vi "Config UserPwd DB.vi"(8 "error in (no error)":errorcluster, 11 "Configuration in":refnum<class "Configuration.lvclass">) -> (0 "error out":errorcluster, 3 "Configuration out":refnum<class "Configuration.lvclass">)   [LabVIEW 2016, in "UserPwd DB.lvlib" / "UserPwd DB Configuration.lvclass"]
uses:
  <userlib>/Common Components/UserPwd DB/UserPwd DB Config/UserPwd DB Configuration.lvclass
  <userlib>/Configuration Dialog Actor/Configuration.lvclass
  <userlib>/Common Components/UserPwd DB/UserPwd DB Config/data row.ctl
  <userlib>/Common Components/UserPwd DB/UserPwd DB Config/Access Level.ctl
  C:/Program Files (x86)/National Instruments/LabVIEW 2016/user.lib/Configuration Dialog Actor/Configuration.lvclass
  <userlib>/Common Components/UserPwd DB/UserPwd DB Config/UserPwd DB Configuration.lvclass/UserPwd DB Configuration.ctl
  <userlib>/Common Components/UserPwd DB/UserPwd DB/Data input.ctl
  <userlib>/Common Components/UserPwd DB/UserPwd DB/Access Level.ctl
  <userlib>/Common Components/UserPwd DB/UserPwd DB/UserPwd DB.lvclass
panel:
  out "Permission Labels":string[](array[string])
  in  "Remove Selected":bool
  in  "New User":bool
  in  "UserPwd Array":T1[](array[typedef]) {"Access Level" items=["Admin"=0, "User"=1, "Guest"=10]}
  in  "Revert":bool
  in  "Apply":bool
  # "Username"
  # "Access Level"
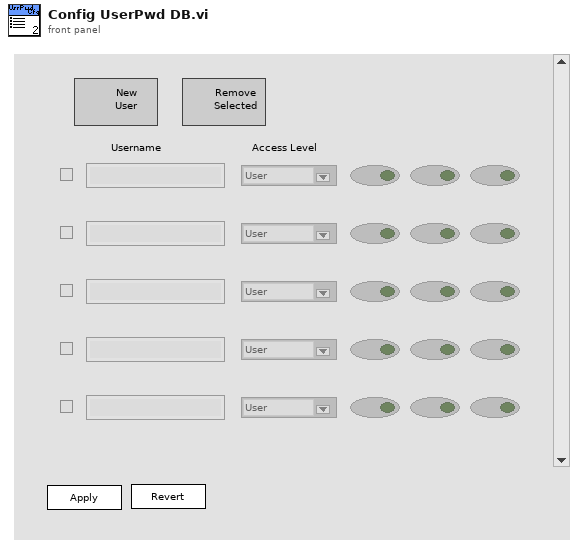
[diagram p1: front panel]
types:
  T1 = typedef "UserPwd DB.lvlib/UserPwd DB Configuration.lvclass/data row.ctl" = cluster{"Checkbox":bool, "Username":string, "Access Level":T2, "Array of Permissions":bool[]}
  T2 = typedef "UserPwd DB.lvlib/UserPwd DB Configuration.lvclass/Access Level.ctl" = u16
  T3 = typedef "UserPwd DB.lvlib/UserPwd DB.lvclass/Data input.ctl" = cluster{"Password":string, "Access":T4, "Array of Permissions":bool[]}
  T4 = typedef "UserPwd DB.lvlib/UserPwd DB.lvclass/Access Level.ctl" = enum16{"Admin", "User lv1", "User lv2", "User lv3", "User lv4", "User lv5", "User lv6", "User lv7", "User lv8", "User lv9", "Guest"}
  T5 = cluster{bool, string, "Access":T4, "2D Array of Permissions":bool[]}
  T6 = cluster{"Checkbox":bool, "Username":bool, "Access Level":bool, "Array of Permissions":bool[]}[]
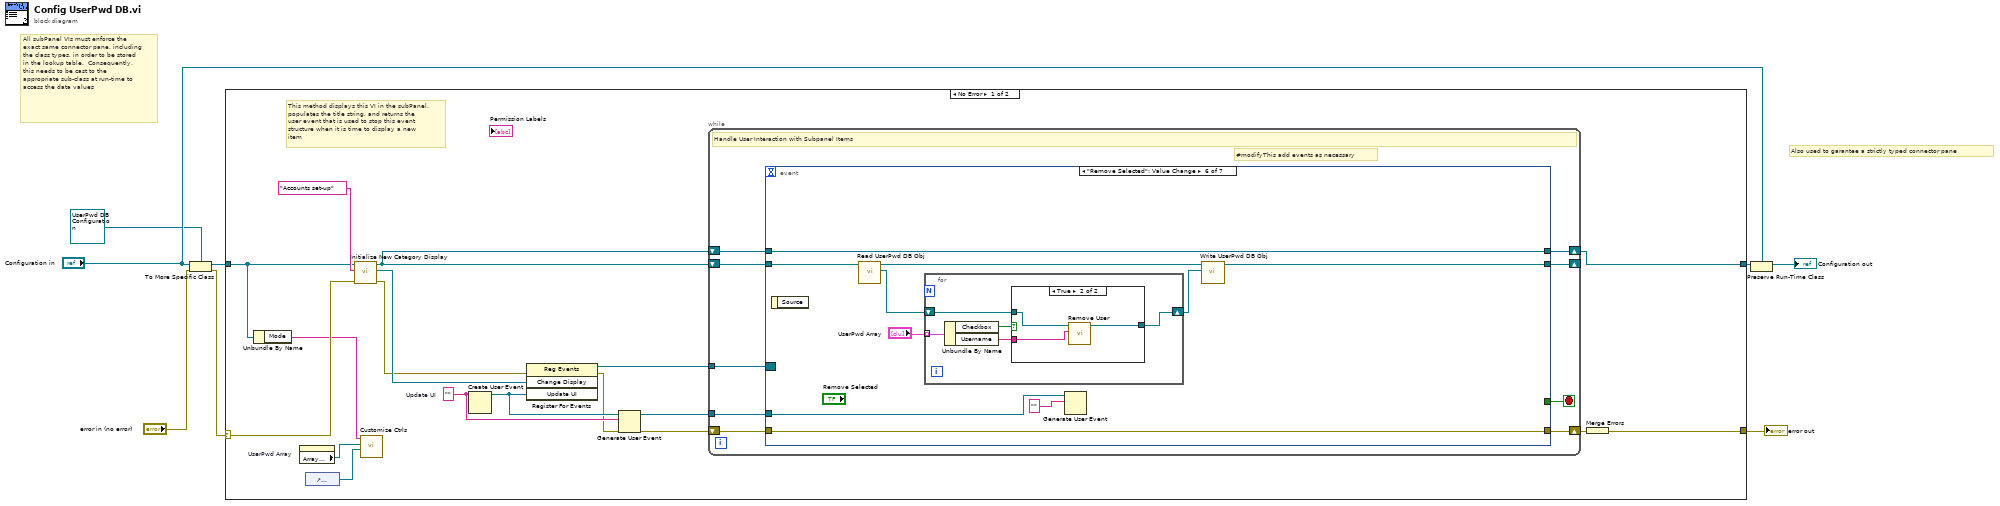
[diagram p0: block diagram]
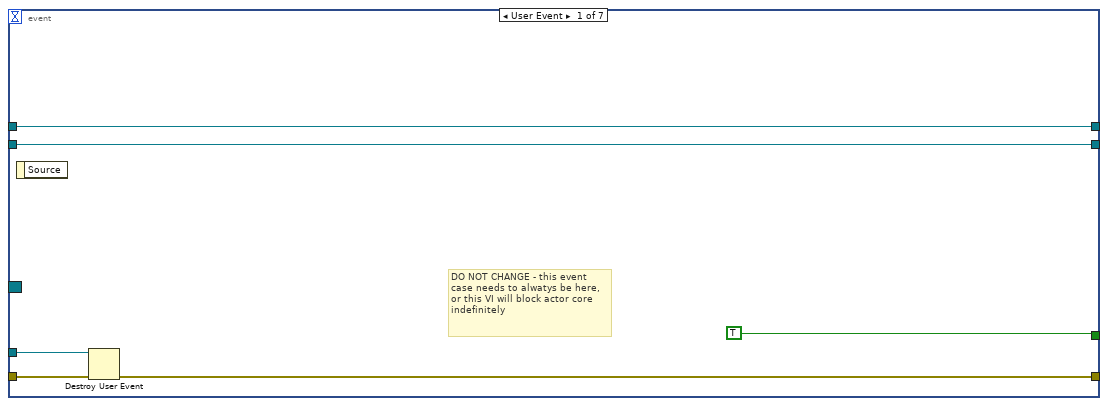
[diagram p2: hidden frame]
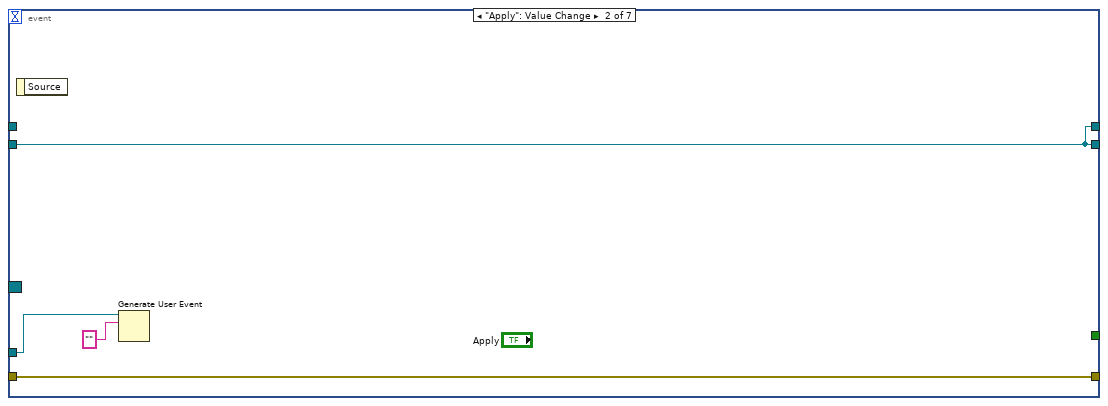
[diagram p3: hidden frame]
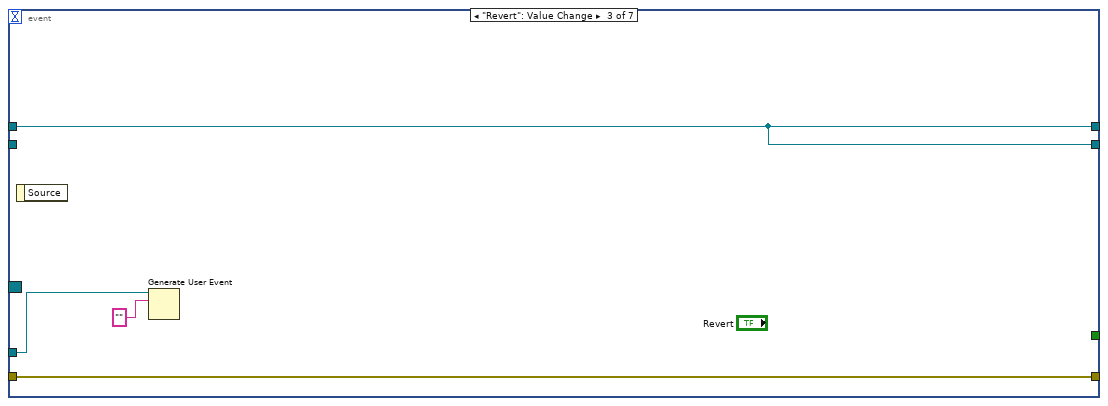
[diagram p4: hidden frame]
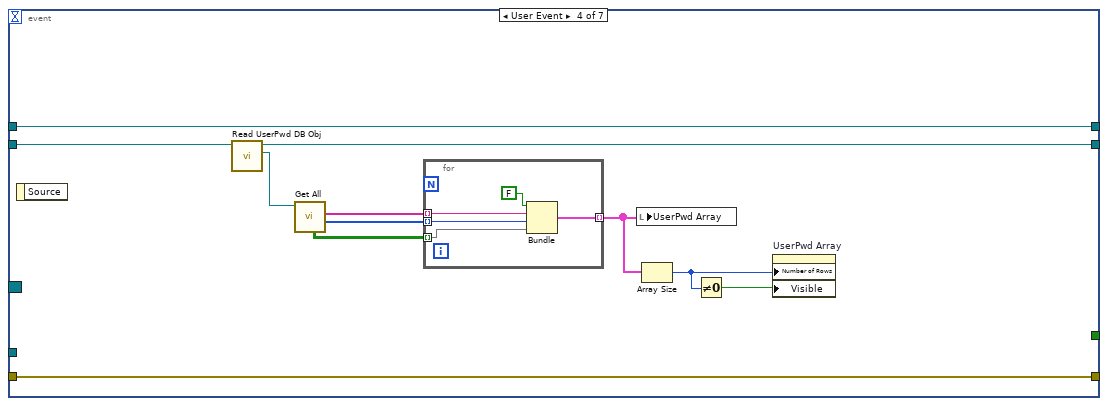
[diagram p5: hidden frame]
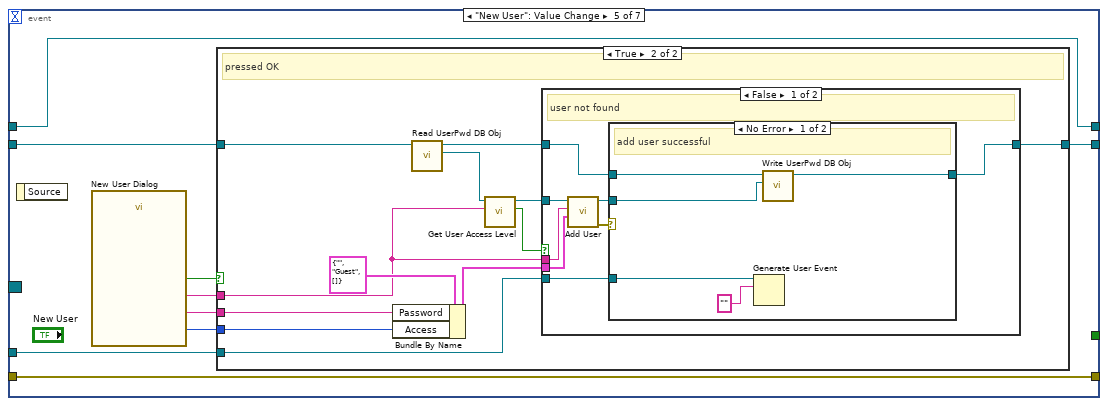
[diagram p6: hidden frame]
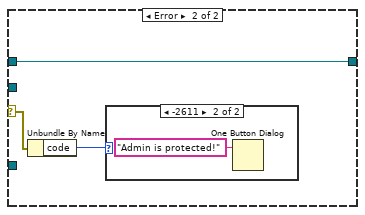
[diagram p8: hidden frame]
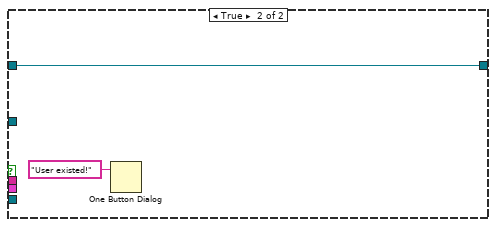
[diagram p10: hidden frame]
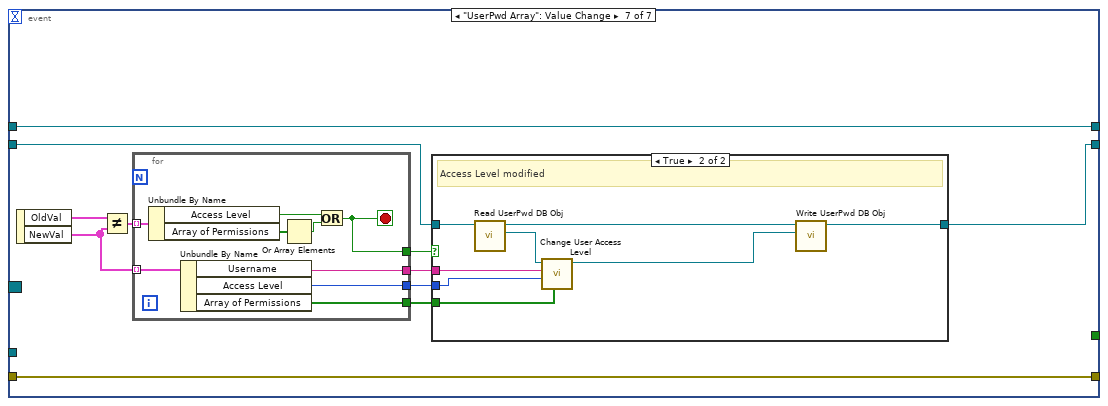
[diagram p12: hidden frame]
diagram:
  # "Also used to garantee a strictly typed connector pane"
  # "All subPanel VIs must enforce the exact same connector pane, including the class types, in order to be stored in the lookup table.  Consequently, this needs to be cast to the appropriate sub-class at run-time to access the data values"
  n1 = To More Specific Class(target class=refnum<class "UserPwd DB Configuration.lvclass"> refnum ("UserPwd DB.lvlib:UserPwd DB Configuration.lvclass"), reference="Configuration in", error in="error in (no error)") -> (specific class reference=w6:refnum<class "UserPwd DB Configuration.lvclass">, error out=w2:errorcluster)
  n2 = case shown="No Error" w2 {
    selector: w2 -> [w24 w155]
    tunnel: w6 -> [w10 w156]
    tunnel: [w17 w156] -> w8
    tunnel: [w26 w155] -> w7
    frame No Error {
      w18 = ""  # Update UI
      # "This method displays this VI in the subPanel, populates the title string, and returns the user event that is used to stop this event structure when it is time to display a new item"
      n3 = Unbundle By Name(w10) -> ("Mode"=w9:string)
      n4 = property on="UserPwd Array" class="Arr (strict)"() -> ("Array Element"=w12:refnum<vi>)  [unwired: 2 in, 2 out]
      n5 = control-ref of="Permission Labels"() -> (w11:refnum<vi>)
      n6 = call <userlib>:"Initialize New Category Display.vi"("error in (no error)"=w24, "Name to Display"="Accounts set-up", "Configuration in"=w10) -> ("error out"=w15:errorcluster, "Change Display"=w23:refnum<user-event>, "Configuration Out"=w20:refnum<class "UserPwd DB Configuration.lvclass">)  [unwired: 6 in]
      n7 = call <userlib>:"Customize Ctrls.vi"("Permission Labels Ref"=w11, "Array Element Ref"=w12, "Mode"=w9) -> ()  [unwired: 8 in, 1 out]
      n8 = Create User Event(user event datatype=w18) -> (user event=w19:refnum<user-event>)  [unwired: 1 in, 1 out]
      n9 = register-events(error in=w15, w23, w19) -> (reference out=w22:refnum<event-registration>, error out=w14:errorcluster)  [unwired: 1 in]
      n10 = Generate User Event(user event=w19, event data cluster=w18, error in=w14) -> (user event out=w16:refnum<user-event>, error out=w13:errorcluster)  [unwired: 1 in]
      n11 = while {
        tunnel: w22 -> [w34]
        shift-right: [w33] -> w21
        shift-left: w13 -> [w32]
        shift-right: [w30] -> _
        shift-left: w20 -> [w31]
        tunnel: w16 -> [w28]
        shift-right: [w27] -> w17
        shift-left: w20 -> [w29]
        stop <- w35 stop-if-true
        # "#modifyThis add events as necessary"
        # "Handle User Interaction with Subpanel Items"
        n12 = event shown="[5] \"Remove Selected\": Value Change" {
          selector: w34 -> [_ _ _ _ _ _ _]
          dyn-events: _ -> [_ _ _ _ _ _ _]
          timeout: _ -> [_ _ _ _ _ _ _]
          tunnel: [TRUE _ _ _ _ _ _] -> w35
          tunnel: [w36 w45 w49 w60 w74 w116 w136] -> w33
          tunnel: w32 -> [w37 w45 w49 w60 w74 w116 w136]
          tunnel: w31 -> [w40 w44 _ w59 w71 w115 w131]
          tunnel: [w40 w44 w48 w58 w72 w110 w130] -> w30
          tunnel: w29 -> [w39 _ w48 w54 w66 w114 w135]
          tunnel: w28 -> [w38 w42 w46 _ w67 w108 _]
          tunnel: [w39 w44 w48 w54 w66 w114 w135] -> w27
          event User Event {
            # "DO NOT CHANGE - this event case needs to alwatys be here, or this VI will block actor core indefinitely"
            n13 = event-data() -> ()  [unwired: 1 in, 1 out]
            n14 = Destroy User Event(user event=w38, error in=w37) -> (error out=w36:errorcluster)
          }
          event "Apply": Value Change {
            n15 = event-data() -> ()  [unwired: 1 in, 1 out]
            n16 = Generate User Event(user event=w42, event data cluster="" ("event data")) -> ()  [unwired: 2 in, 2 out]
          }
          event "Revert": Value Change {
            n17 = event-data() -> ()  [unwired: 1 in, 1 out]
            n18 = Generate User Event(user event=w46, event data cluster="" ("event data")) -> ()  [unwired: 2 in, 2 out]
          }
          event User Event {
            n19 = event-data() -> ()  [unwired: 1 in, 1 out]
            n20 = call <userlib>:"Read UserPwd DB Obj.vi"("UserPwd DB Configuration in"=w59) -> ("UserPwd DB.lvlib:UserPwd DB.lvclass"=w55:refnum<class "UserPwd DB.lvclass">, "UserPwd DB Configuration out"=w58:refnum<class "UserPwd DB Configuration.lvclass">)  [unwired: 9 in]
            n21 = call <userlib>:"Get All.vi"("UserPwd DB in"=w55) -> ("Access Levels"=w56:T4[], "Usernames"=w57:string[], "2D Array of Permissions"=w50:bool[][])  [unwired: 6 in, 2 out]
            n22 = for {
              tunnel: w57 -> [w65] mode=indexing
              tunnel: w56 -> [w64] mode=indexing
              tunnel: [w63] -> w53 mode=indexing
              tunnel: w50 -> [w61] mode=indexing
              n23 = Bundle(FALSE, w65, "Access"=w64, "2D Array of Permissions"=w61) -> (w63:T5)  [unwired: 1 in]
            }
            n24 = local write "UserPwd Array"(w53) -> ()
            n25 = Array Size(array=w53) -> (size(s)=w52:i32)
            n26 = Not Equal To 0?(x=w52) -> (x != 0?=w51:bool)
            n27 = property on="UserPwd Array" class="Arr (strict)"("Number of Rows"=w52, "Visible"=w51) -> ()  [unwired: 2 in, 2 out]
          }
          event "New User": Value Change {
            n28 = event-data() -> ()  [unwired: 1 in, 1 out]
            n29 = call <userlib>:"New User Dialog.vi"() -> ("Access Level"=w70:T2, "Password"=w69:string, "Username"=w68:string, "OK"=w73:bool)  [unwired: 15 in, 1 out]
            n30 = case shown="True" w73 {
              tunnel: [w75 w76] -> w72
              tunnel: w71 -> [w75 w87]
              tunnel: w70 -> [_ w84]
              tunnel: w69 -> [_ w82]
              tunnel: w68 -> [_ w79]
              tunnel: w67 -> [_ w78]
              frame False {
              }
              frame True {
                # "pressed OK"
                n31 = Bundle By Name(cluster=T3 {"Password"="", "Access"=enum."Guest", "Array of Permissions"=[]} ("Data"), "Password"=w82, "Access"=w84) -> (w83:T3)
                n32 = call <userlib>:"Read UserPwd DB Obj.vi"("UserPwd DB Configuration in"=w87) -> ("UserPwd DB.lvlib:UserPwd DB.lvclass"=w86:refnum<class "UserPwd DB.lvclass">, "UserPwd DB Configuration out"=w77:refnum<class "UserPwd DB Configuration.lvclass">)  [unwired: 9 in]
                n33 = call <userlib>:"Get User Access Level.vi"("Username"=w79, "UserPwd DB in"=w86) -> ("found"=w80:bool, "UserPwd DB out"=w81:refnum<class "UserPwd DB.lvclass">)  [unwired: 5 in, 3 out]
                n34 = case shown="False" w80 {
                  tunnel: w83 -> [w95 _]
                  tunnel: w79 -> [w94 _]
                  tunnel: w81 -> [w93 _]
                  tunnel: w78 -> [w92 _]
                  tunnel: w77 -> [w91 w105]
                  tunnel: [w90 w105] -> w76
                  frame False {
                    # "user not found"
                    n35 = call <userlib>:"Add User.vi"("Data"=w95, "Username"=w94, "UserPwd DB in"=w93) -> ("error out"=w89:errorcluster, "UserPwd DB out"=w88:refnum<class "UserPwd DB.lvclass">)  [unwired: 7 in]
                    n36 = case shown="No Error" w89 {
                      selector: w89 -> [_ w103]
                      tunnel: w92 -> [w97 _]
                      tunnel: w91 -> [w99 w101]
                      tunnel: [w98 w101] -> w90
                      tunnel: w88 -> [w96 _]
                      frame No Error {
                        # "add user successful"
                        n37 = Generate User Event(user event=w97, event data cluster="" ("event data")) -> ()  [unwired: 2 in, 2 out]
                        n38 = call <userlib>:"Write UserPwd DB Obj.vi"("UserPwd DB.lvlib:UserPwd DB.lvclass"=w96, "UserPwd DB Configuration in"=w99) -> ("UserPwd DB Configuration out"=w98:refnum<class "UserPwd DB Configuration.lvclass">)  [unwired: 9 in]
                      }
                      frame Error {
                        n39 = Unbundle By Name(w103) -> ("code"=w102:i32)
                        n40 = case shown="-2611" w102 {
                          frame Default {
                          }
                          frame -2611 {
                            n41 = One Button Dialog(message="Admin is protected!") -> ()  [unwired: 1 in, 1 out]
                          }
                        }
                      }
                    }
                  }
                  frame True {
                    n42 = One Button Dialog(message="User existed!") -> ()  [unwired: 1 in, 1 out]
                  }
                }
              }
            }
          }
          event "Remove Selected": Value Change {
            n43 = event-data() -> ()  [unwired: 1 in, 1 out]
            n44 = call <userlib>:"Read UserPwd DB Obj.vi"("UserPwd DB Configuration in"=w115) -> ("UserPwd DB.lvlib:UserPwd DB.lvclass"=w111:refnum<class "UserPwd DB.lvclass">, "UserPwd DB Configuration out"=w112:refnum<class "UserPwd DB Configuration.lvclass">)  [unwired: 9 in]
            n45 = for {
              tunnel: "UserPwd Array" -> [w121] mode=indexing
              shift-right: [w119] -> w109
              shift-left: w111 -> [w120]
              n46 = Unbundle By Name(w121) -> ("Checkbox"=w118:bool, "Username"=w117:string)
              n47 = case shown="True" w118 {
                tunnel: w120 -> [w122 w125]
                tunnel: [w122 w124] -> w119
                tunnel: w117 -> [_ w123]
                frame False {
                }
                frame True {
                  n48 = call <userlib>:"Remove User.vi"("Username"=w123, "UserPwd DB in"=w125) -> ("UserPwd DB out"=w124:refnum<class "UserPwd DB.lvclass">)  [unwired: 7 in, 2 out]
                }
              }
            }
            n49 = Generate User Event(user event=w108, event data cluster="" ("event data")) -> ()  [unwired: 2 in, 2 out]
            n50 = call <userlib>:"Write UserPwd DB Obj.vi"("UserPwd DB.lvlib:UserPwd DB.lvclass"=w109, "UserPwd DB Configuration in"=w112) -> ("UserPwd DB Configuration out"=w110:refnum<class "UserPwd DB Configuration.lvclass">)  [unwired: 9 in]
          }
          event "UserPwd Array": Value Change {
            n51 = event-data() -> ("OldVal"=w132:T1[], "NewVal"=w128:T1[])  [unwired: 1 in]
            n52 = Not Equal?(x=w132, y=w128) -> (x != y?=w134:T6)
            n53 = for {
              tunnel: w134 -> [w154] mode=indexing
              tunnel: [w149] -> w133
              tunnel: w128 -> [w152] mode=indexing
              tunnel: [w151] -> w129
              tunnel: [w150] -> w127
              tunnel: [w146] -> w126
              stop <- w149 stop-if-true
              n54 = Unbundle By Name(w154) -> ("Access Level"=w153:bool, "Array of Permissions"=w148:bool[])
              n55 = Unbundle By Name(w152) -> ("Username"=w151:string, "Access Level"=w150:T2, "Array of Permissions"=w146:bool[])
              n56 = Or Array Elements(Boolean array=w148) -> (logical OR=w147:bool)
              n57 = Or(x=w153, y=w147) -> (x .or. y?=w149:bool)
            }
            n58 = case shown="True" w133 {
              tunnel: w131 -> [w137 w145]
              tunnel: [w137 w142] -> w130
              tunnel: w129 -> [_ w140]
              tunnel: w127 -> [_ w139]
              tunnel: w126 -> [_ w138]
              frame False {
              }
              frame True {
                # "Access Level modified"
                n59 = call <userlib>:"Read UserPwd DB Obj.vi"("UserPwd DB Configuration in"=w145) -> ("UserPwd DB.lvlib:UserPwd DB.lvclass"=w143:refnum<class "UserPwd DB.lvclass">, "UserPwd DB Configuration out"=w144:refnum<class "UserPwd DB Configuration.lvclass">)  [unwired: 9 in]
                n60 = call <userlib>:"Change User Access Level.vi"("Array of Permissions"=w138, "Access"=w139, "Username"=w140, "UserPwd DB in"=w143) -> ("UserPwd DB out"=w141:refnum<class "UserPwd DB.lvclass">)  [unwired: 5 in, 2 out]
                n61 = call <userlib>:"Write UserPwd DB Obj.vi"("UserPwd DB.lvlib:UserPwd DB.lvclass"=w141, "UserPwd DB Configuration in"=w144) -> ("UserPwd DB Configuration out"=w142:refnum<class "UserPwd DB Configuration.lvclass">)  [unwired: 9 in]
              }
            }
          }
        }
      }
      n62 = Merge Errors(w21) -> (w26:errorcluster)
    }
    frame Error {
    }
  }
  "error out" <- w7
  n63 = Preserve Run-Time Class(object in=w8, 2:"Configuration in") -> (object out=→"Configuration out":refnum<class "Configuration.lvclass">)  [unwired: 1 in, 1 out]
